vi "PicoScope4000aGetRapidBlock.vi"(0 "error in":errorcluster, 3 "handle in":i16, 4 "Enabled array":i16[](array[numeric]), 5 "Rapid Block Acquisition Settings":T1) -> (6 "Channel A Buffer":i16[][](array[numeric]), 7 "Channel E Buffer":i16[][](array[numeric]), 8 "Channel B Buffer":i16[][](array[numeric]), 9 "Channel F Buffer":i16[][](array[numeric]), 10 "Channel C Buffer":i16[][](array[numeric]), 11 "Channel G Buffer":i16[][](array[numeric]), 12 "Channel D Buffer":i16[][](array[numeric]), 13 "Channel H Buffer":i16[][](array[numeric]), 14 "error out":errorcluster, 15 "handle out":i16)   [LabVIEW 2009]
doc: "This VI gets a set of blocks captured using rapid block mode. It outputs two-dimensional arrays for each channel that contain data from all the requested captures."
uses:
  ps4000A.dll
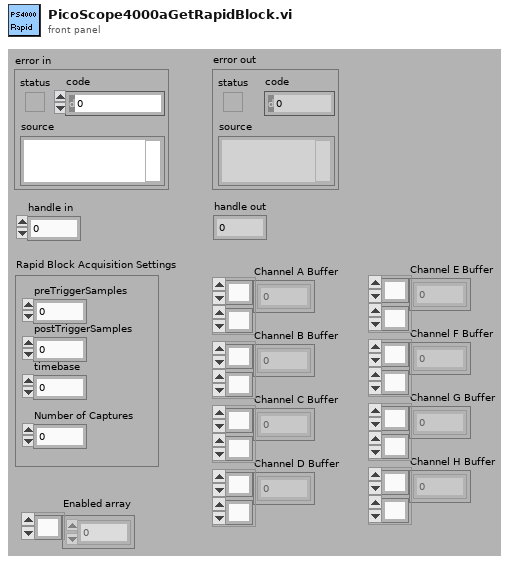
[diagram p1: front panel]
types:
  T1 = cluster{"preTriggerSamples":i32, "postTriggerSamples":i32, "timebase":u32, "Number of Captures":u32}
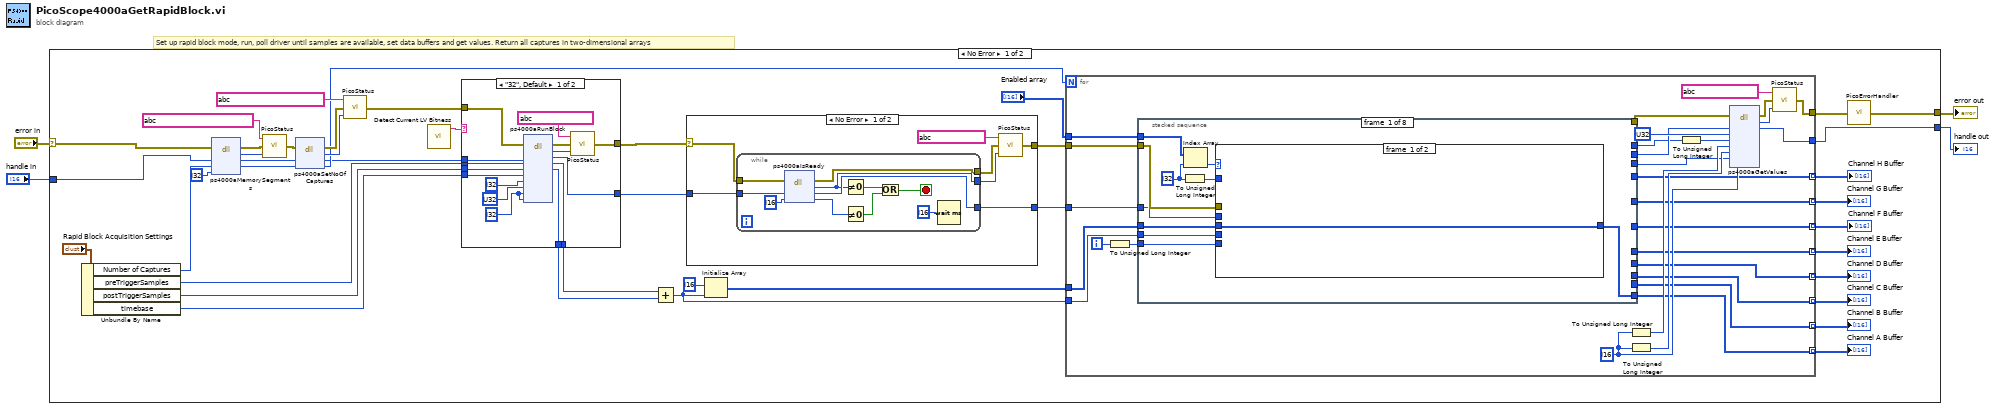
[diagram p0: block diagram]
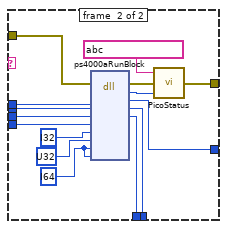
[diagram p2: hidden frame]
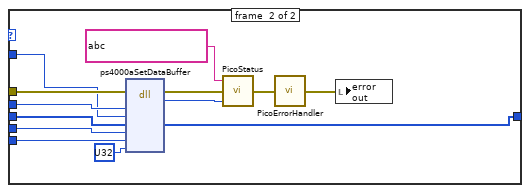
[diagram p3: hidden frame]
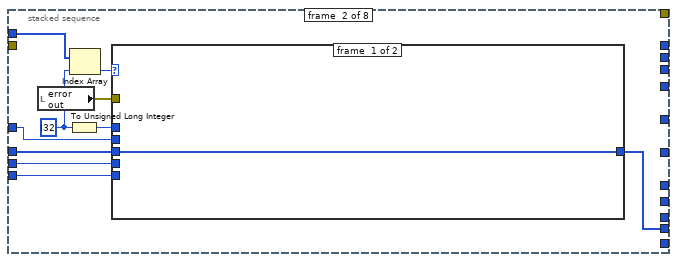
[diagram p4: hidden frame]
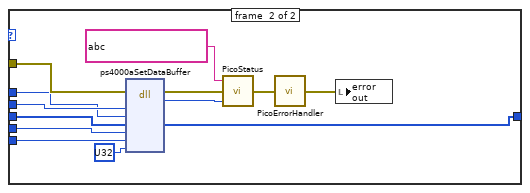
[diagram p5: hidden frame]
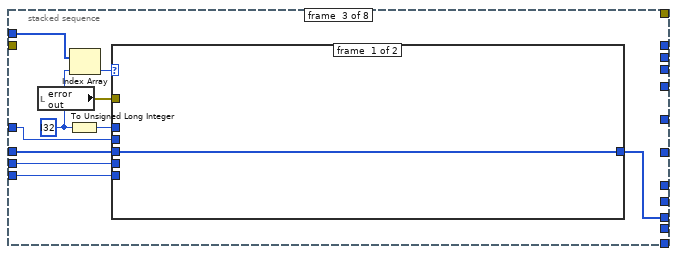
[diagram p6: hidden frame]
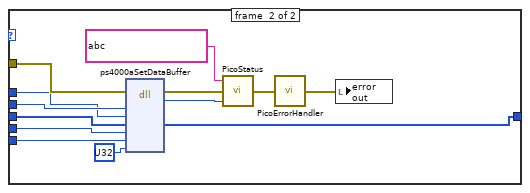
[diagram p7: hidden frame]
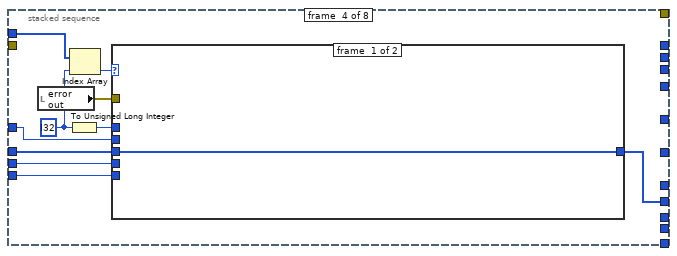
[diagram p8: hidden frame]
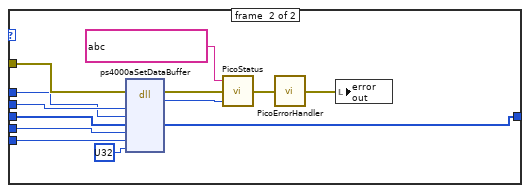
[diagram p9: hidden frame]
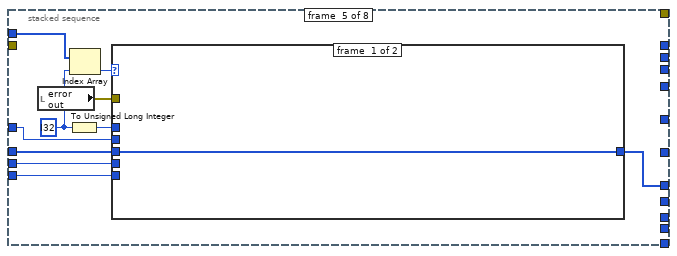
[diagram p10: hidden frame]
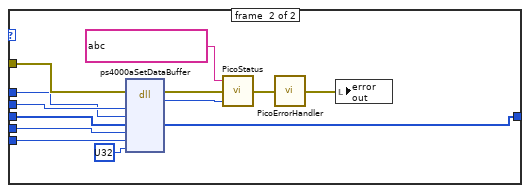
[diagram p11: hidden frame]
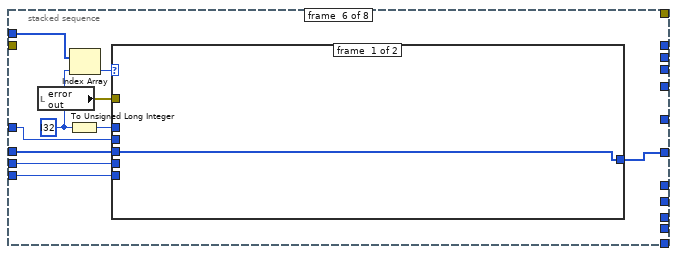
[diagram p12: hidden frame]
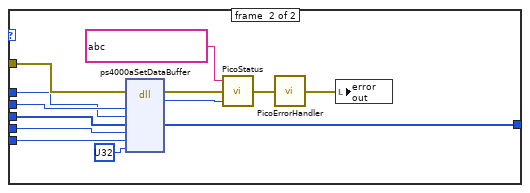
[diagram p13: hidden frame]
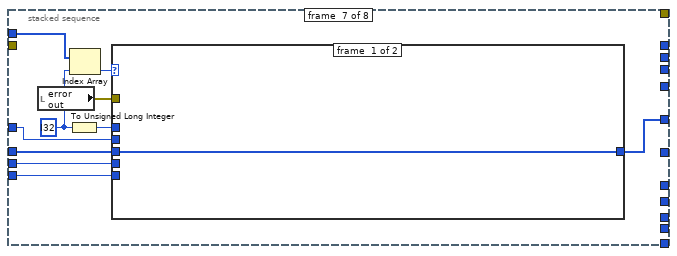
[diagram p14: hidden frame]
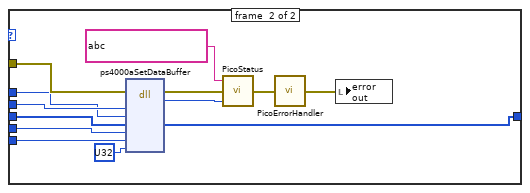
[diagram p15: hidden frame]
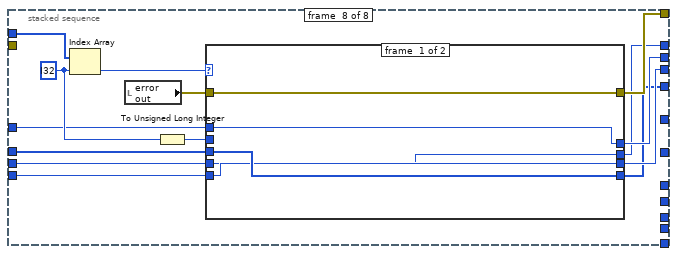
[diagram p16: hidden frame]
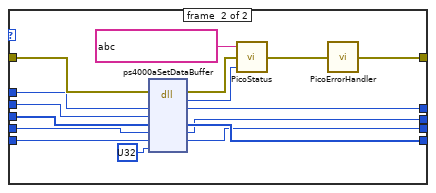
[diagram p17: hidden frame]
diagram:
  # "Set up rapid block mode, run, poll driver until samples are available, set data buffers and get values. Return all captures in two-dimensional arrays"
  n1 = case shown="No Error" "error in" {
    selector: "error in" -> [w36 w330]
    tunnel: [w14 w330] -> w3
    tunnel: "handle in" -> [w35 w329]
    tunnel: [w16 w329] -> w1
    frame #0 {
      n2 = Unbundle By Name("Rapid Block Acquisition Settings") -> ("Number of Captures"=w31:u32, "preTriggerSamples"=w39:i32, "postTriggerSamples"=w38:i32, "timebase"=w40:u32)
      n3 = dll-call lib="ps4000a.dll" fn="ps4000aMemorySegments" ("ps3000.dll:_ps3000_open_unit@0")(error in=w36, "handle"=w35, "nSegments"=w31, "nMaxSamples"=i32 ?) -> (error out=w33:errorcluster, "PICO_STATUS"=w34:u32, "handle"=w28:i16, "nSegments"=w29:u32)  [unwired: 3 in, 1 out]
      n4 = call "PicoStatus.vi"("PICO STATUS"=w34, "error in"=w33, "source"=string ?) -> ("error out"=w27:errorcluster)
      n5 = dll-call lib="ps4000a.dll" fn="ps4000aSetNoOfCaptures" ("ps3000.dll:_ps3000_open_unit@0")(error in=w27, "handle"=w28, "nCaptures"=w29) -> (error out=w25:errorcluster, "PICO_STATUS"=w26:u32, "handle"=w21:i16, "nCaptures"=w22:u32)  [unwired: 2 in, 1 out]
      n6 = call "PicoStatus.vi"("PICO STATUS"=w26, "error in"=w25, "source"=string ?) -> ("error out"=w23:errorcluster)
      n7 = call "Detect Current LV Bitness.vi"() -> ("bitness"=w5:string)  [unwired: 11 in]
      n8 = case shown="\"32\", Default" w5 {
        tunnel: [w61 w76] -> w46
        tunnel: [w60 w75] -> w44
        tunnel: [w59 w74] -> w43
        tunnel: w40 -> [w58 w73]
        tunnel: w39 -> [w57 w72]
        tunnel: w38 -> [w56 w71]
        tunnel: [w53 w68] -> w37
        tunnel: w23 -> [w51 w66]
        tunnel: w21 -> [w50 w65]
        frame #0 {
          w47 = i32 ? ("pParameter")
          n9 = dll-call lib="ps4000A.dll" fn="ps4000aRunBlock" ("ps3000.dll:_ps3000_open_unit@0")(error in=w51, "handle"=w50, "preTriggerSamples"=w57, "postTriggerSamples"=w56, "timebase"=w58, "timeindisposedMs"=i32 ? ("pParameter"), "segmentIndex"=u32 ? ("pParameter"), "lpReady"=w47, "pParameter"=w47) -> (error out=w54:errorcluster, "PICO_STATUS"=w55:u32, "handle"=w61:i16, "preTriggerSamples"=w60:i32, "postTriggerSamples"=w59:i32)  [unwired: 7 in, 1 out]
          n10 = call "PicoStatus.vi"("PICO STATUS"=w55, "error in"=w54, "source"=string ?) -> ("error out"=w53:errorcluster)
        }
        frame #1 {
          w62 = i64 ? ("pParameter")
          n11 = dll-call lib="ps4000A.dll" fn="ps4000aRunBlock" ("ps3000.dll:_ps3000_open_unit@0")(error in=w66, "handle"=w65, "preTriggerSamples"=w72, "postTriggerSamples"=w71, "timebase"=w73, "timeindisposedMs"=i32 ? ("pParameter"), "segmentIndex"=u32 ? ("pParameter"), "lpReady"=w62, "pParameter"=w62) -> (error out=w69:errorcluster, "PICO_STATUS"=w70:u32, "handle"=w76:i16, "preTriggerSamples"=w75:i32, "postTriggerSamples"=w74:i32)  [unwired: 7 in, 1 out]
          n12 = call "PicoStatus.vi"("PICO STATUS"=w70, "error in"=w69, "source"=string ?) -> ("error out"=w68:errorcluster)
        }
      }
      n13 = Add(x=w44, y=w43) -> (x+y=w11:i32)
      n14 = case shown="No Error" w37 {
        selector: w37 -> [w313 w327]
        tunnel: w46 -> [w315 w328]
        tunnel: [w314 w328] -> w45
        tunnel: [w312 w327] -> w42
        frame #0 {
          n15 = while {
            tunnel: [w326] -> w314
            tunnel: w315 -> [w325]
            tunnel: [w320] -> w310
            tunnel: w313 -> [w319]
            tunnel: [w318] -> w311
            stop <- w324 stop-if-true
            n16 = dll-call lib="ps4000a.dll" fn="ps4000aIsReady" ("ps3000.dll:_ps3000_open_unit@0")(error in=w319, "handle"=w325, "ready"=i16 ?) -> (error out=w318:errorcluster, "PICO_STATUS"=w320:u32, "handle"=w326:i16, "ready"=w321:i16)  [unwired: 2 in, 1 out]
            n17 = Not Equal To 0?(x=w320) -> (x != 0?=w322:bool)
            n18 = Not Equal To 0?(x=w321) -> (x != 0?=w323:bool)
            n19 = Or(x=w322, y=w323) -> (x .or. y?=w324:bool)
            n20 = Wait (ms)(milliseconds to wait=i16 ? ("ready")) -> ()  [unwired: 1 out]
          }
          n21 = call "PicoStatus.vi"("PICO STATUS"=w310, "error in"=w311, "source"=string ?) -> ("error out"=w312:errorcluster)
        }
        frame #1 {
        }
      }
      n22 = Initialize Array(i16 ? ("element"), w11) -> (w10:i16[])
      n23 = for {
        N: w22 -> [_]
        tunnel: w45 -> [w94]
        tunnel: w42 -> [w96]
        tunnel: [w86] -> w20 mode=indexing
        tunnel: [w87] -> w19 mode=indexing
        tunnel: [w88] -> w18 mode=indexing
        tunnel: [w89] -> w17 mode=indexing
        tunnel: w11 -> [w90]
        tunnel: [w100] -> w16
        tunnel: [w99] -> w15
        tunnel: "Enabled array" -> [w95]
        tunnel: w10 -> [w93]
        tunnel: [w85] -> w9 mode=indexing
        tunnel: [w81] -> w8 mode=indexing
        tunnel: [w80] -> w7 mode=indexing
        tunnel: [w79] -> w6 mode=indexing
        i -> [w92]
        w105 = i16 ? ("overflow")
        n24 = To Unsigned Long Integer(number=w92) -> (unsigned 32bit integer=w91:u32)
        n25 = stacked-sequence {
          tunnel: [w113 _ _ _ _ _ _ _] -> w89
          tunnel: w95 -> [w115 w139 w163 w187 w211 w235 w259 w287]
          tunnel: w96 -> [w110 _ _ _ _ _ _ _]
          tunnel: w94 -> [w109 w135 w159 w183 w207 w231 w255 w283]
          tunnel: w93 -> [w108 w134 w158 w182 w206 w230 w254 w282]
          tunnel: w91 -> [w107 w133 w157 w181 w205 w229 w253 w281]
          tunnel: w90 -> [w106 w132 w156 w180 w204 w228 w252 w280]
          tunnel: [_ w131 _ _ _ _ _ _] -> w88
          tunnel: [_ _ w155 _ _ _ _ _] -> w87
          tunnel: [_ _ _ w178 _ _ _ _] -> w86
          tunnel: [_ _ _ _ w202 _ _ _] -> w85
          tunnel: [_ _ _ _ _ _ _ w278] -> w84
          tunnel: [_ _ _ _ _ _ _ w277] -> w83
          tunnel: [_ _ _ _ _ _ _ w276] -> w82
          tunnel: [_ _ _ _ _ _ _ w275] -> w81
          tunnel: [_ _ _ _ _ _ w250 _] -> w80
          tunnel: [_ _ _ _ _ w226 _ _] -> w79
          tunnel: [_ _ _ _ _ _ _ w274] -> w78
          frame #0 {
            w112 = i32 ? ("index")
            n26 = To Unsigned Long Integer(number=w112) -> (unsigned 32bit integer=w111:u32)
            n27 = Index Array(array=w115, index=w112) -> (element=w114:i16)
            n28 = case shown="1" w114 {
              tunnel: w110 -> [_ w126]
              tunnel: w109 -> [_ w125]
              tunnel: w108 -> [w116 w119]
              tunnel: [w116 w124] -> w113
              tunnel: w111 -> [_ w121]
              tunnel: w107 -> [_ w118]
              tunnel: w106 -> [_ w117]
              frame #0 {
              }
              frame #1 {
                n29 = dll-call lib="ps4000a.dll" fn="ps4000aSetDataBuffer" ("ps3000.dll:_ps3000_open_unit@0")(error in=w126, "handle"=w125, "channel"=w121, "buffer"=w119, "bufferLth"=w117, "segmentIndex"=w118, "mode"=u32 ?) -> (error out=w129:errorcluster, "PICO_STATUS"=w128:u32, "buffer"=w124:i16[])  [unwired: 7 in, 1 out]
                n30 = call "PicoStatus.vi"("PICO STATUS"=w128, "error in"=w129, "source"=string ?) -> ("error out"=w123:errorcluster)
                n31 = call "PicoErrorHandler.vi"("error in"=w123) -> ("error out"=w120:errorcluster)
                n32 = local write "error out"(w120) -> ()
              }
            }
          }
          frame #1 {
            w137 = i32 ? ("index")
            n33 = local read "error out"() -> (w130:errorcluster)
            n34 = To Unsigned Long Integer(number=w137) -> (unsigned 32bit integer=w136:u32)
            n35 = Index Array(array=w139, index=w137) -> (element=w138:i16)
            n36 = case shown="1" w138 {
              tunnel: w130 -> [_ w150]
              tunnel: w135 -> [_ w149]
              tunnel: w134 -> [w140 w143]
              tunnel: [w140 w148] -> w131
              tunnel: w136 -> [_ w145]
              tunnel: w133 -> [_ w142]
              tunnel: w132 -> [_ w141]
              frame #0 {
              }
              frame #1 {
                n37 = dll-call lib="ps4000a.dll" fn="ps4000aSetDataBuffer" ("ps3000.dll:_ps3000_open_unit@0")(error in=w150, "handle"=w149, "channel"=w145, "buffer"=w143, "bufferLth"=w141, "segmentIndex"=w142, "mode"=u32 ?) -> (error out=w153:errorcluster, "PICO_STATUS"=w152:u32, "buffer"=w148:i16[])  [unwired: 7 in, 1 out]
                n38 = call "PicoStatus.vi"("PICO STATUS"=w152, "error in"=w153, "source"=string ?) -> ("error out"=w147:errorcluster)
                n39 = call "PicoErrorHandler.vi"("error in"=w147) -> ("error out"=w144:errorcluster)
                n40 = local write "error out"(w144) -> ()
              }
            }
          }
          frame #2 {
            w161 = i32 ? ("index")
            n41 = local read "error out"() -> (w154:errorcluster)
            n42 = To Unsigned Long Integer(number=w161) -> (unsigned 32bit integer=w160:u32)
            n43 = Index Array(array=w163, index=w161) -> (element=w162:i16)
            n44 = case shown="1" w162 {
              tunnel: w154 -> [_ w174]
              tunnel: w159 -> [_ w173]
              tunnel: w158 -> [w164 w167]
              tunnel: [w164 w172] -> w155
              tunnel: w160 -> [_ w169]
              tunnel: w157 -> [_ w166]
              tunnel: w156 -> [_ w165]
              frame #0 {
              }
              frame #1 {
                n45 = dll-call lib="ps4000a.dll" fn="ps4000aSetDataBuffer" ("ps3000.dll:_ps3000_open_unit@0")(error in=w174, "handle"=w173, "channel"=w169, "buffer"=w167, "bufferLth"=w165, "segmentIndex"=w166, "mode"=u32 ?) -> (error out=w177:errorcluster, "PICO_STATUS"=w176:u32, "buffer"=w172:i16[])  [unwired: 7 in, 1 out]
                n46 = call "PicoStatus.vi"("PICO STATUS"=w176, "error in"=w177, "source"=string ?) -> ("error out"=w171:errorcluster)
                n47 = call "PicoErrorHandler.vi"("error in"=w171) -> ("error out"=w168:errorcluster)
                n48 = local write "error out"(w168) -> ()
              }
            }
          }
          frame #3 {
            w185 = i32 ? ("index")
            n49 = local read "error out"() -> (w179:errorcluster)
            n50 = To Unsigned Long Integer(number=w185) -> (unsigned 32bit integer=w184:u32)
            n51 = Index Array(array=w187, index=w185) -> (element=w186:i16)
            n52 = case shown="1" w186 {
              tunnel: w179 -> [_ w198]
              tunnel: w183 -> [_ w197]
              tunnel: w182 -> [w188 w191]
              tunnel: [w188 w196] -> w178
              tunnel: w184 -> [_ w193]
              tunnel: w181 -> [_ w190]
              tunnel: w180 -> [_ w189]
              frame #0 {
              }
              frame #1 {
                n53 = dll-call lib="ps4000a.dll" fn="ps4000aSetDataBuffer" ("ps3000.dll:_ps3000_open_unit@0")(error in=w198, "handle"=w197, "channel"=w193, "buffer"=w191, "bufferLth"=w189, "segmentIndex"=w190, "mode"=u32 ?) -> (error out=w201:errorcluster, "PICO_STATUS"=w200:u32, "buffer"=w196:i16[])  [unwired: 7 in, 1 out]
                n54 = call "PicoStatus.vi"("PICO STATUS"=w200, "error in"=w201, "source"=string ?) -> ("error out"=w195:errorcluster)
                n55 = call "PicoErrorHandler.vi"("error in"=w195) -> ("error out"=w192:errorcluster)
                n56 = local write "error out"(w192) -> ()
              }
            }
          }
          frame #4 {
            w209 = i32 ? ("index")
            n57 = local read "error out"() -> (w203:errorcluster)
            n58 = To Unsigned Long Integer(number=w209) -> (unsigned 32bit integer=w208:u32)
            n59 = Index Array(array=w211, index=w209) -> (element=w210:i16)
            n60 = case shown="1" w210 {
              tunnel: w203 -> [_ w222]
              tunnel: w207 -> [_ w221]
              tunnel: w206 -> [w212 w215]
              tunnel: [w212 w220] -> w202
              tunnel: w208 -> [_ w217]
              tunnel: w205 -> [_ w214]
              tunnel: w204 -> [_ w213]
              frame #0 {
              }
              frame #1 {
                n61 = dll-call lib="ps4000A.dll" fn="ps4000aSetDataBuffer" ("ps3000.dll:_ps3000_open_unit@0")(error in=w222, "handle"=w221, "channel"=w217, "buffer"=w215, "bufferLth"=w213, "segmentIndex"=w214, "mode"=u32 ?) -> (error out=w225:errorcluster, "PICO_STATUS"=w224:u32, "buffer"=w220:i16[])  [unwired: 7 in, 1 out]
                n62 = call "PicoStatus.vi"("PICO STATUS"=w224, "error in"=w225, "source"=string ?) -> ("error out"=w219:errorcluster)
                n63 = call "PicoErrorHandler.vi"("error in"=w219) -> ("error out"=w216:errorcluster)
                n64 = local write "error out"(w216) -> ()
              }
            }
          }
          frame #5 {
            w233 = i32 ? ("index")
            n65 = local read "error out"() -> (w227:errorcluster)
            n66 = To Unsigned Long Integer(number=w233) -> (unsigned 32bit integer=w232:u32)
            n67 = Index Array(array=w235, index=w233) -> (element=w234:i16)
            n68 = case shown="1" w234 {
              tunnel: w227 -> [_ w246]
              tunnel: w231 -> [_ w245]
              tunnel: w230 -> [w236 w239]
              tunnel: [w236 w244] -> w226
              tunnel: w232 -> [_ w241]
              tunnel: w229 -> [_ w238]
              tunnel: w228 -> [_ w237]
              frame #0 {
              }
              frame #1 {
                n69 = dll-call lib="ps4000a.dll" fn="ps4000aSetDataBuffer" ("ps3000.dll:_ps3000_open_unit@0")(error in=w246, "handle"=w245, "channel"=w241, "buffer"=w239, "bufferLth"=w237, "segmentIndex"=w238, "mode"=u32 ?) -> (error out=w249:errorcluster, "PICO_STATUS"=w248:u32, "buffer"=w244:i16[])  [unwired: 7 in, 1 out]
                n70 = call "PicoStatus.vi"("PICO STATUS"=w248, "error in"=w249, "source"=string ?) -> ("error out"=w243:errorcluster)
                n71 = call "PicoErrorHandler.vi"("error in"=w243) -> ("error out"=w240:errorcluster)
                n72 = local write "error out"(w240) -> ()
              }
            }
          }
          frame #6 {
            w257 = i32 ? ("index")
            n73 = local read "error out"() -> (w251:errorcluster)
            n74 = To Unsigned Long Integer(number=w257) -> (unsigned 32bit integer=w256:u32)
            n75 = Index Array(array=w259, index=w257) -> (element=w258:i16)
            n76 = case shown="1" w258 {
              tunnel: w251 -> [_ w270]
              tunnel: w255 -> [_ w269]
              tunnel: w254 -> [w260 w263]
              tunnel: [w260 w268] -> w250
              tunnel: w256 -> [_ w265]
              tunnel: w253 -> [_ w262]
              tunnel: w252 -> [_ w261]
              frame #0 {
              }
              frame #1 {
                n77 = dll-call lib="ps4000a.dll" fn="ps4000aSetDataBuffer" ("ps3000.dll:_ps3000_open_unit@0")(error in=w270, "handle"=w269, "channel"=w265, "buffer"=w263, "bufferLth"=w261, "segmentIndex"=w262, "mode"=u32 ?) -> (error out=w273:errorcluster, "PICO_STATUS"=w272:u32, "buffer"=w268:i16[])  [unwired: 7 in, 1 out]
                n78 = call "PicoStatus.vi"("PICO STATUS"=w272, "error in"=w273, "source"=string ?) -> ("error out"=w267:errorcluster)
                n79 = call "PicoErrorHandler.vi"("error in"=w267) -> ("error out"=w264:errorcluster)
                n80 = local write "error out"(w264) -> ()
              }
            }
          }
          frame #7 {
            w285 = i32 ? ("index")
            n81 = Index Array(array=w287, index=w285) -> (element=w286:i16)
            n82 = local read "error out"() -> (w279:errorcluster)
            n83 = To Unsigned Long Integer(number=w285) -> (unsigned 32bit integer=w284:u32)
            n84 = case shown="1" w286 {
              tunnel: w279 -> [w291 w305]
              tunnel: w283 -> [w290 w304]
              tunnel: w282 -> [w292 w299]
              tunnel: [w292 w303] -> w275
              tunnel: w284 -> [_ w300]
              tunnel: w281 -> [w289 w298]
              tunnel: w280 -> [w288 w297]
              tunnel: [w291 w296] -> w278
              tunnel: [w290 w295] -> w277
              tunnel: [w289 w294] -> w276
              tunnel: [w288 w293] -> w274
              frame #0 {
              }
              frame #1 {
                n85 = dll-call lib="ps4000A.dll" fn="ps4000aSetDataBuffer" ("ps3000.dll:_ps3000_open_unit@0")(error in=w305, "handle"=w304, "channel"=w300, "buffer"=w299, "bufferLth"=w297, "segmentIndex"=w298, "mode"=u32 ?) -> (error out=w308:errorcluster, "PICO_STATUS"=w307:u32, "handle"=w295:i16, "buffer"=w303:i16[], "bufferLth"=w293:i32, "segmentIndex"=w294:u32)  [unwired: 4 in, 1 out]
                n86 = call "PicoStatus.vi"("PICO STATUS"=w307, "error in"=w308, "source"=string ?) -> ("error out"=w302:errorcluster)
                n87 = call "PicoErrorHandler.vi"("error in"=w302) -> ("error out"=w296:errorcluster)
              }
            }
          }
        }
        n88 = To Unsigned Long Integer(number=w105) -> (unsigned 32bit integer=w98:u32)
        n89 = To Unsigned Long Integer(number=w105) -> (unsigned 32bit integer=w97:u32)
        n90 = To Unsigned Long Integer(number=w78) -> (unsigned 32bit integer=w77:u32)
        n91 = dll-call lib="ps4000a.dll" fn="ps4000aGetValues" ("ps3000.dll:_ps3000_open_unit@0")(error in=w84, "handle"=w83, "startIndex"=u32 ?, "noOfSamples"=w77, "downSampleRatio"=w98, "downSampleRatioMode"=w97, "segmentIndex"=w82, "overflow"=w105) -> (error out=w102:errorcluster, "PICO_STATUS"=w101:u32, "handle"=w100:i16)  [unwired: 8 in, 1 out]
        n92 = call "PicoStatus.vi"("PICO STATUS"=w101, "error in"=w102, "source"=string ?) -> ("error out"=w99:errorcluster)
      }
      "Channel D Buffer" <- w20
      "Channel C Buffer" <- w19
      "Channel B Buffer" <- w18
      "Channel A Buffer" <- w17
      "Channel H Buffer" <- w8
      "Channel G Buffer" <- w7
      "Channel F Buffer" <- w6
      "Channel E Buffer" <- w9
      n93 = call "PicoErrorHandler.vi"("error in"=w15) -> ("error out"=w14:errorcluster)
    }
    frame #1 {
    }
  }
  "error out" <- w3
  "handle out" <- w1
